vi "G#Object_GetObjectGraph.vi"(5 "error in (no error)":errorcluster) -> (15 "all refs":refnum<class "G#Object.lvclass">[](array[class]), 16 "dependent objects":cluster{refnum<class "G#Object.lvclass">[]}[](array[cluster]), 19 "error out":errorcluster)   [LabVIEW 2017, in "G#Object.lvclass"]
doc: "Returns all objects and there corresponding dependent objects. This forms the object dependency graph."
uses:
  G#Object.lvclass
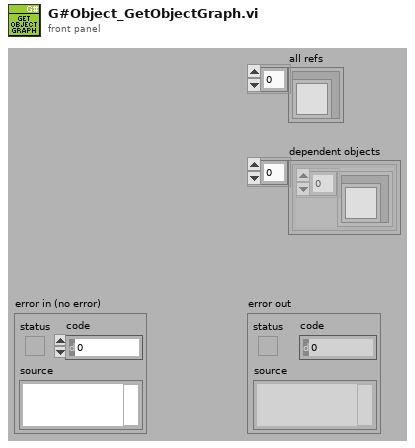
[diagram p1: front panel]
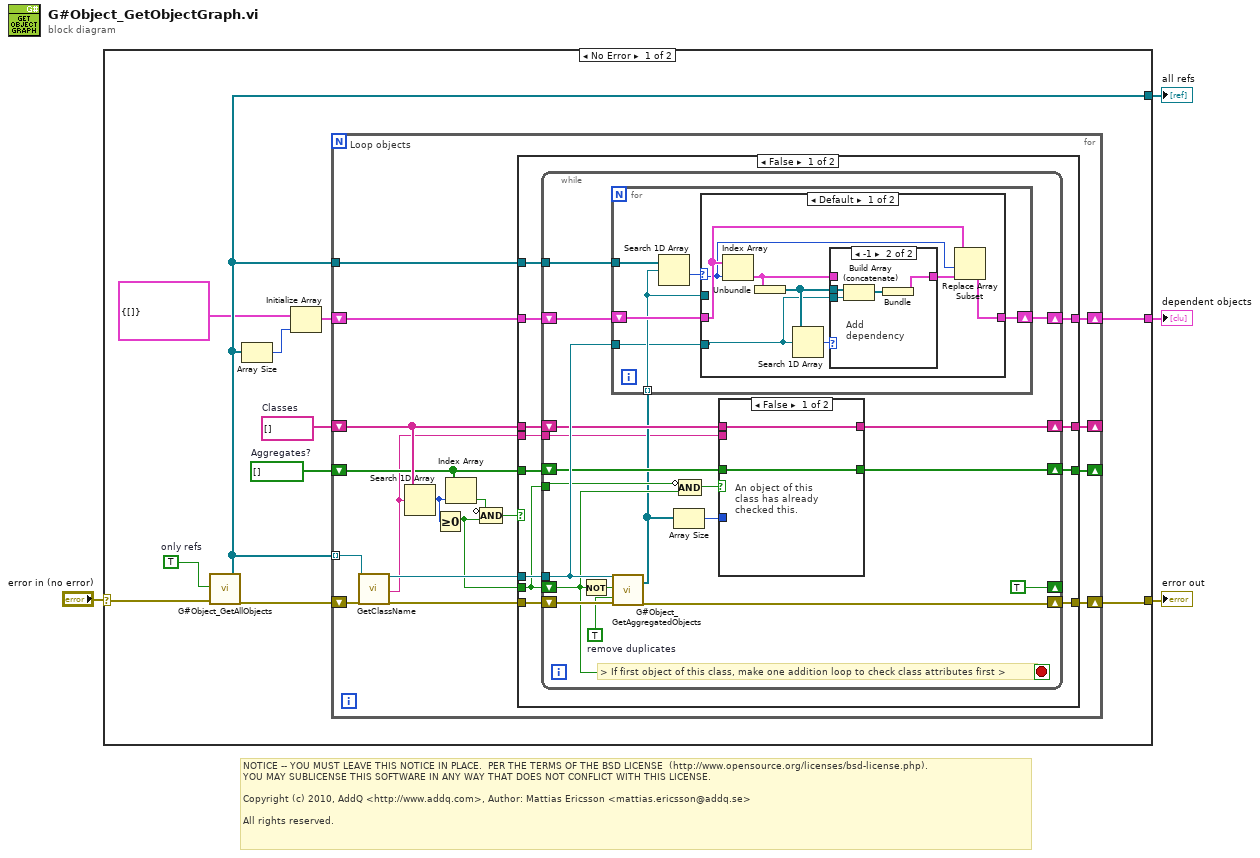
[diagram p0: block diagram]
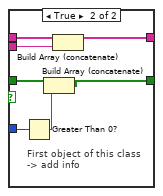
[diagram p2: hidden frame]
diagram:
  # "NOTICE -- YOU MUST LEAVE THIS NOTICE IN PLACE.  PER THE TERMS OF THE BSD LICENSE  (http://www.opensource.org/licenses/bsd-license.php).\nYOU MAY SUBLICENSE THIS SOFTWARE IN ANY WAY THAT DOES NOT CONFLICT WITH THIS LICENSE.\n\nCopyright (c) 2010, AddQ <http://www.addq.com>, Author: Mattias Ericsson <mattias.ericsson@addq.se>\n\nAll rights reserved."
  n1 = case shown="No Error" "error in (no error)" {
    selector: "error in (no error)" -> [w15 w97]
    tunnel: [w11 w97] -> w3
    tunnel: [w8 _] -> w2
    tunnel: [w10 _] -> w1
    frame No Error {
      w9 = TRUE  # only refs
      w12 = bool[] []  # Aggregates?
      w13 = string[] []  # Classes
      n2 = call "G#Object_GetAllObjects.vi"("only refs (F)"=w9, "error in (no error)"=w15) -> ("all refs"=w8:refnum<class "G#Object.lvclass">[], "error out"=w14:errorcluster)  [unwired: 14 in, 2 out]
      n3 = Array Size(array=w8) -> (size(s)=w7:i32)
      n4 = Initialize Array(cluster{refnum<class "G#Object.lvclass">[]} {[]}, w7) -> (w6:cluster{refnum<class "G#Object.lvclass">[]}[])
      n5 = for {
        shift-right: [w19] -> w11
        shift-left: w14 -> [w32]
        tunnel: w8 -> [w30] mode=indexing
        shift-right: [w21] -> _
        shift-left: w13 -> [w24]
        shift-right: [w20] -> _
        shift-left: w12 -> [w23]
        shift-right: [w22] -> w10
        shift-left: w6 -> [w25]
        tunnel: w8 -> [w16]
        # "Loop objects"
        n6 = call-dynamic "GetClassName.vi"("reference in"=w30, "error in (no error)"=w32) -> ("reference out"=w29:refnum<class "G#Object.lvclass">, "full class name"=w17:string, "error out"=w31:errorcluster)  [unwired: 13 in, 2 out]
        n7 = Search 1D Array(1D array=w24, element=w17) -> (index of element=w28:i32)  [unwired: 1 in]
        n8 = Greater Or Equal To 0?(x=w28) -> (x >= 0?=w18:bool)
        n9 = Index Array(array=w23, index=w28) -> (element=w27:bool)
        n10 = Compound Arithmetic op=AND(invert w27, w18) -> (w26:bool)
        n11 = case shown="False" w26 {
          tunnel: w31 -> [w44 w93]
          tunnel: w29 -> [w43 _]
          tunnel: w16 -> [w33 _]
          tunnel: w25 -> [w42 w96]
          tunnel: w24 -> [w41 w95]
          tunnel: w23 -> [w40 w94]
          tunnel: [w34 w96] -> w22
          tunnel: [w36 w95] -> w21
          tunnel: [w35 w94] -> w20
          tunnel: [w39 w93] -> w19
          tunnel: w18 -> [w38 _]
          tunnel: w17 -> [w37 _]
          frame False {
            n12 = while {
              tunnel: w43 -> [w59]
              shift-right: [w58] -> w34
              shift-left: w42 -> [w60]
              shift-right: [w49] -> w36
              shift-left: w41 -> [w57]
              shift-right: [w48] -> w35
              shift-left: w40 -> [w56]
              shift-right: [TRUE] -> _
              shift-left: w38 -> [w54]
              shift-right: [w61] -> w39
              shift-left: w44 -> [w63]
              tunnel: w38 -> [w55]
              tunnel: w37 -> [w50]
              tunnel: w33 -> [w47]
              stop <- w54 stop-if-true
              w46 = TRUE  # remove duplicates
              # "> If first object of this class, make one addition loop to check class attributes first >"
              n13 = Not(x=w54) -> (.not. x?=w45:bool)
              n14 = call "G#Object_GetAggregatedObjects.vi"("reference in"=w59, "class attributes (F)"=w45, "remove duplicates (F)"=w46, "error in (no error)"=w63) -> ("aggregated objects"=w52:refnum<class "G#Object.lvclass">[], "error out"=w61:errorcluster)  [unwired: 12 in, 2 out]
              n15 = for {
                shift-right: [w74] -> w58
                shift-left: w60 -> [w77]
                tunnel: w52 -> [w76] mode=indexing
                tunnel: w59 -> [w75]
                tunnel: w47 -> [w73]
                n16 = Search 1D Array(1D array=w73, element=w76) -> (index of element=w78:i32)  [unwired: 1 in]
                n17 = case shown="Default" w78 {
                  selector: w78 -> [w84 _]
                  tunnel: w77 -> [w86 w92]
                  tunnel: w76 -> [_ _]
                  tunnel: w75 -> [w81 _]
                  tunnel: [w85 w92] -> w74
                  frame Default {
                    n18 = Index Array(array=w86, index=w84) -> (element=w80:cluster{refnum<class "G#Object.lvclass">[]})
                    n19 = Unbundle(w80) -> (w82:refnum<class "G#Object.lvclass">[])
                    n20 = Search 1D Array(1D array=w82, element=w81) -> (index of element=w83:i32)  [unwired: 1 in]
                    n21 = case shown="-1" w83 {
                      tunnel: w82 -> [_ w91]
                      tunnel: w81 -> [_ w90]
                      tunnel: w80 -> [w87 _]
                      tunnel: [w87 w88] -> w79
                      frame Default {
                        # "Already\nadded"
                      }
                      frame -1 {
                        # "Add\ndependency"
                        n22 = Build Array (concatenate)(w91, w90) -> (w89:refnum<class "G#Object.lvclass">[])
                        n23 = Bundle(w89) -> (w88:cluster{refnum<class "G#Object.lvclass">[]})  [unwired: 1 in]
                      }
                    }
                    n24 = Replace Array Subset(array=w86, new element=w79, index=w84) -> (w85:cluster{refnum<class "G#Object.lvclass">[]}[])
                  }
                  frame -1 {
                    # "It must be an invalid reference that has been\naggregated"
                  }
                }
              }
              n25 = Array Size(array=w52) -> (size(s)=w51:i32)
              n26 = Compound Arithmetic op=AND(invert w55, w54) -> (w53:bool)
              n27 = case shown="False" w53 {
                tunnel: w57 -> [w65 w71]
                tunnel: w56 -> [w64 w68]
                tunnel: w51 -> [_ w72]
                tunnel: w50 -> [_ w69]
                tunnel: [w65 w70] -> w49
                tunnel: [w64 w66] -> w48
                frame False {
                  # "An object of this\nclass has already\nchecked this."
                }
                frame True {
                  # "First object of this class\n-> add info"
                  n28 = Greater Than 0?(x=w72) -> (x > 0?=w67:bool)
                  n29 = Build Array (concatenate)(w68, w67) -> (w66:bool[])
                  n30 = Build Array (concatenate)(w71, w69) -> (w70:string[])
                }
              }
            }
          }
          frame True {
            # "Objects from this class has been tested before and this class\ndoesn't contain any aggregates."
          }
        }
      }
    }
    frame Error {
    }
  }
  "error out" <- w3
  "all refs" <- w2
  "dependent objects" <- w1
